vi "Dictionary Create__ogtk.vi"(8 "error in (no error)":errorcluster, 10 "initial dictionary (empty)":cluster{"key":variant, "value":variant}[](array[cluster])) -> (0 "error out":errorcluster, 3 "dictionary out":T1)   [LabVIEW 2012]
doc: "Creates a new instance of empty dictionary data and returns a dictionary reference associated with the newly created dictionary."
uses:
  <userlib>/_OpenG.lib/dictionary/dictionary.llb/Dictionary Data__ogtk.ctl
  <userlib>/_OpenG.lib/dictionary/dictionary.llb/Dictionary Object RefNum__ogtk.ctl
  <userlib>/_OpenG.lib/dictionary/dictionary.llb/Dictionary Object RefNum - Enum__ogtk.ctl
panel:
  in  "Data in":T2
  # "Dictionary Create.vi\n\nCreates a new instance of empty dictionary data and returns a dictionary reference associated with the newly created dictionary.\n\nPlease visit http://www.OpenG.org to learn about the\nOpen Source LabVIEW software movement.\n\nNOTICE -- YOU MUST LEAVE THIS NOTICE IN PLACE.  PER THE TERMS OF THE LICENSE BELOW, YOU MAY SUBLICENSE THIS SOFTWARE \nIN ANY WAY THAT DOES NOT CONFLICT WITH THIS LICENSE.\n\n### BSD License (http://www.opensource.org/licenses/bsd-license.php) Begin ###\n \nCopyright (c) 2005, Jim Kring <jim@jimkring.com>\n\nAll rights reserved.\n\nRedistribution and use in source and binary forms, with or without modification, are permitted provided that the following conditions are met:\n\n    * Redistributions of source code must retain the above copyright notice, this list of conditions and the following disclaimer.\n    * Redistributions in binary form must reproduce the above copyright notice, this list of conditions and the following disclaimer in the \n       documentation and/or other materials provided with the distribution.\n    * Neither the name of SciWare, James Kring, Inc., nor the names of its contributors may be used to endorse or promote products derived \n       from this software without specific prior written permission.\n\nTHIS SOFTWARE IS PROVIDED BY THE COPYRIGHT HOLDERS AND CONTRIBUTORS \"AS IS\" AND ANY EXPRESS OR IMPLIED WARRANTIES, \nINCLUDING, BUT NOT LIMITED TO, THE IMPLIED WARRANTIES OF MERCHANTABILITY AND FITNESS FOR A PARTICULAR PURPOSE ARE \nDISCLAIMED. IN NO EVENT SHALL THE COPYRIGHT OWNER OR CONTRIBUTORS BE LIABLE FOR ANY DIRECT, INDIRECT, INCIDENTAL,\n SPECIAL, EXEMPLARY, OR CONSEQUENTIAL DAMAGES (INCLUDING, BUT NOT LIMITED TO, PROCUREMENT OF SUBSTITUTE GOODS OR \nSERVICES; LOSS OF USE, DATA, OR PROFITS; OR BUSINESS INTERRUPTION) HOWEVER CAUSED AND ON ANY THEORY OF LIABILITY, \nWHETHER IN CONTRACT, STRICT LIABILITY, OR TORT (INCLUDING NEGLIGENCE OR OTHERWISE) ARISING IN ANY WAY OUT OF THE USE \nOF THIS SOFTWARE, EVEN IF ADVISED OF THE POSSIBILITY OF SUCH DAMAGE.\n\n### BSD License End ###"
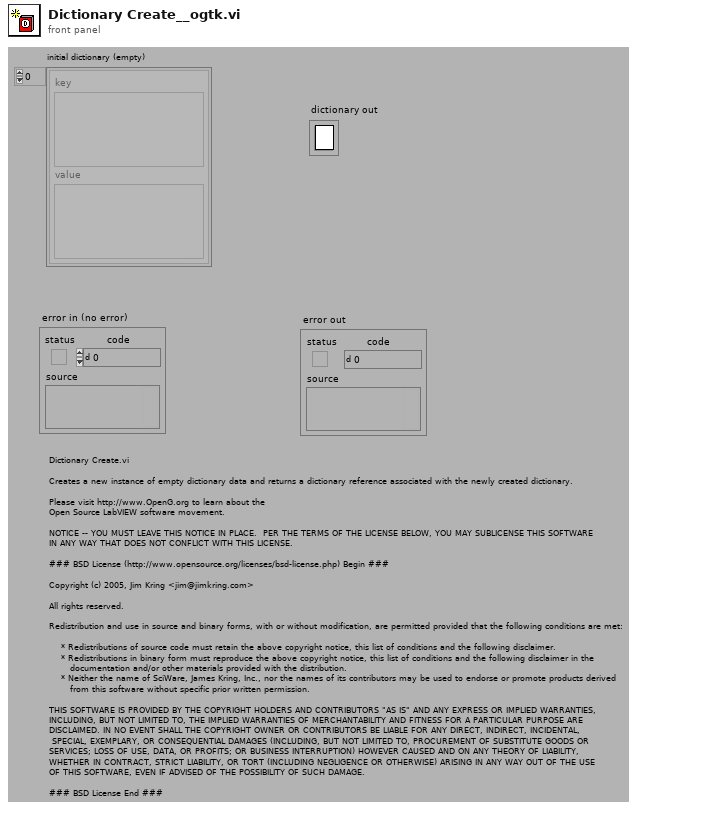
[diagram p1: front panel]
types:
  T1 = typedef "Dictionary Object RefNum__ogtk.ctl" = refnum<k1>
  T2 = typedef "Dictionary Data__ogtk.ctl" = cluster{"keys":variant[], "values":variant[]}
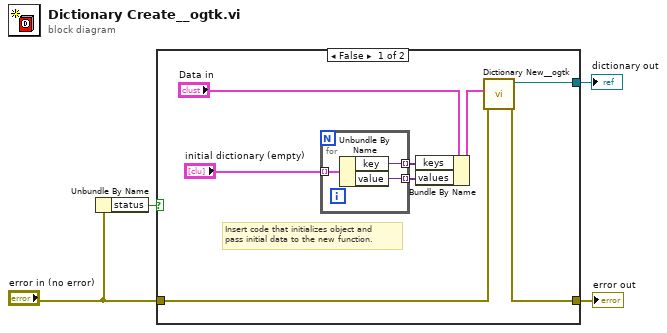
[diagram p0: block diagram]
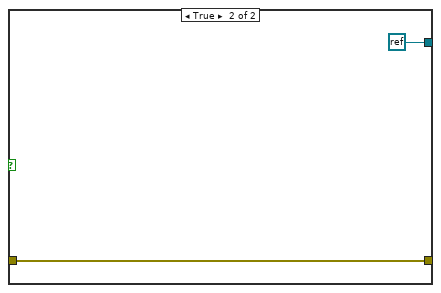
[diagram p2: hidden frame]
diagram:
  n1 = Unbundle By Name("error in (no error)") -> ("status"=w4:bool)
  n2 = case shown="False" w4 {
    tunnel: "error in (no error)" -> [w12 w17]
    tunnel: [w11 w17] -> w2
    tunnel: [w10 refnum<k0> refnum] -> w1
    frame False {
      # "Insert code that initializes object and\npass initial data to the new function."
      n3 = for {
        tunnel: "initial dictionary (empty)" -> [w15] mode=indexing
        tunnel: [w14] -> w7 mode=indexing
        tunnel: [w13] -> w8 mode=indexing
        n4 = Unbundle By Name(w15) -> ("key"=w14:variant, "value"=w13:variant)
      }
      n5 = Bundle By Name(cluster="Data in", "keys"=w7, "values"=w8) -> (w6:T2)
      n6 = call <userlib>:"Dictionary New__ogtk.vi"("error in (no error)"=w12, "Data in"=w6) -> ("error out"=w11:errorcluster, "Object RefNum"=w10:T1)  [unwired: 8 in]
    }
    frame True {
    }
  }
  "error out" <- w2
  "dictionary out" <- w1
